vi "Find optimal frequency.vi"(6 "Bottom end of range (GHz) (140.0)":dbl=140.0, 7 "Top end of range (GHz) (141.0)":dbl=141.0, 8 "Find optimal for negative polarization?":bool, 9 "C":dbl, 10 "Fit parameters":T2={"A"=0.572086, "S"=0.0835606, "M1"=140.286, "M2"=140.486}, 11 "Physical constants":T1={"T1e (s)"=0.03, "T1n (s)"=1500.0}) -> (2 "Steady state at optimal frequency":dbl, 3 "Optimal frequency (GHz)":dbl)   [LabVIEW 2018]
uses:
  Fit Parameters.ctl
  Physical Constants.ctl
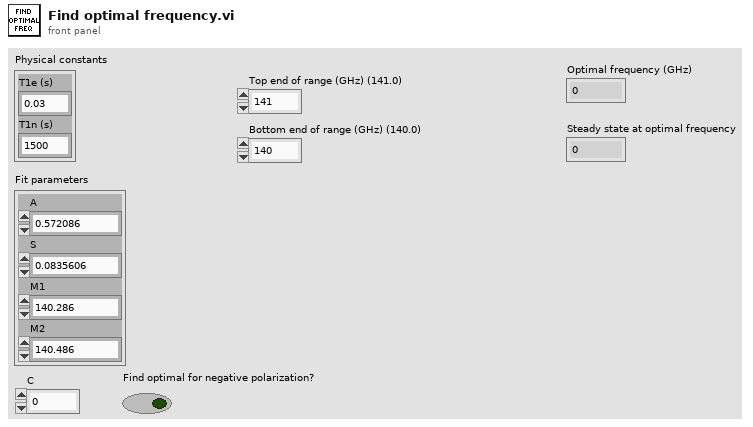
[diagram p1: front panel]
types:
  T1 = typedef "Physical Constants.ctl" = cluster{"T1e (s)":dbl, "T1n (s)":dbl}
  T2 = typedef "Fit Parameters.ctl" = cluster{"A":dbl, "S":dbl, "M1":dbl, "M2":dbl}
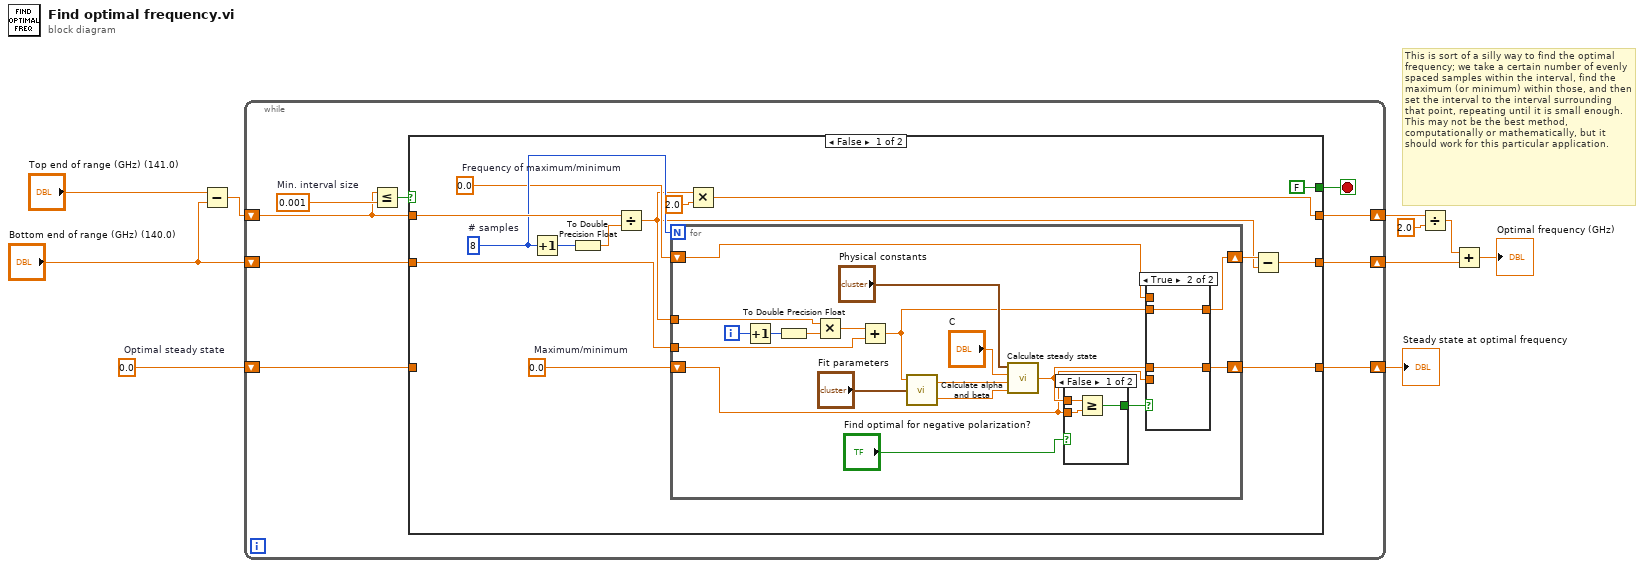
[diagram p0: block diagram]
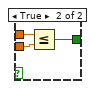
[diagram p3: hidden frame]
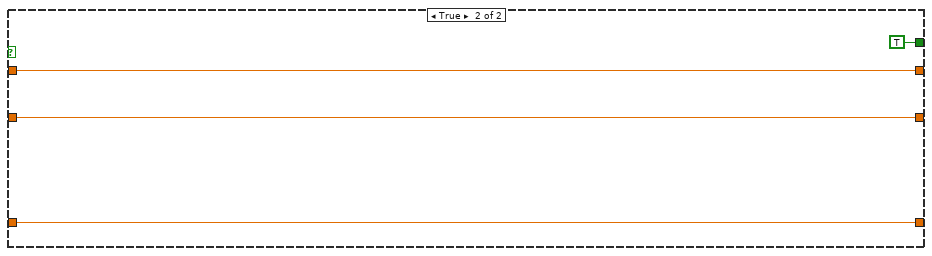
[diagram p4: hidden frame]
diagram:
  w2 = 0.0  # Optimal steady state
  # "This is sort of a silly way to find the optimal frequency; we take a certain number of evenly spaced samples within the interval, find the maximum (or minimum) within those, and then set the interval to the interval surrounding that point, repeating until it is small enough.  This may not be the best method, computationally or mathematically, but it should work for this particular application."
  n1 = Subtract(x="Top end of range (GHz) (141.0)", y="Bottom end of range (GHz) (140.0)") -> (x-y=w8:dbl)
  n2 = while {
    shift-right: [w15] -> w7
    shift-left: w8 -> [w16]
    shift-right: [w13] -> w4
    shift-left: "Bottom end of range (GHz) (140.0)" -> [w14]
    shift-right: [w12] -> w1
    shift-left: w2 -> [w11]
    stop <- w17 stop-if-true
    w19 = 0.001  # Min. interval size
    n3 = Less Or Equal?(x=w16, y=w19) -> (x <= y?=w18:bool)
    n4 = case shown="False" w18 {
      tunnel: [FALSE TRUE] -> w17
      tunnel: w16 -> [w32 w64]
      tunnel: [w27 w64] -> w15
      tunnel: w14 -> [w24 w65]
      tunnel: [w21 w65] -> w13
      tunnel: [w20 w63] -> w12
      tunnel: w11 -> [_ w63]
      frame False {
        w25 = 0.0  # Maximum/minimum
        w26 = 0.0  # Frequency of maximum/minimum
        w29 = 8  # # samples
        n5 = Increment(x=w29) -> (x+1=w30:i32)
        n6 = To Double Precision Float(number=w30) -> (double precision float=w31:dbl)
        n7 = Divide(x=w32, y=w31) -> (x/y=w22:dbl)
        n8 = for {
          N: w29 -> [_]
          tunnel: w22 -> [w51]
          shift-right: [w37] -> w23
          shift-left: w26 -> [w35]
          shift-right: [w36] -> w20
          shift-left: w25 -> [w34]
          tunnel: w24 -> [w39]
          i -> [w49]
          n9 = Increment(x=w49) -> (x+1=w50:i32)
          n10 = To Double Precision Float(number=w50) -> (double precision float=w52:dbl)
          n11 = Multiply(x=w51, y=w52) -> (x*y=w40:dbl)
          n12 = Add(x=w40, y=w39) -> (x+y=w38:dbl)
          n13 = call "Calculate alpha and beta.vi"("Fit parameters"="Fit parameters", "Frequency (GHz)"=w38) -> ("Beta"=w45:dbl, "Alpha"=w46:dbl)  [unwired: 1 in]
          n14 = call "Calculate steady state.vi"("Beta"=w45, "Alpha"=w46, "C"="C", "Physical constants"="Physical constants") -> ("Steady state"=w41:dbl)
          n15 = case shown="False" "Find optimal for negative polarization?" {
            tunnel: w41 -> [w59 w62]
            tunnel: w34 -> [w58 w61]
            tunnel: [w57 w60] -> w42
            frame False {
              n16 = Greater Or Equal?(x=w59, y=w58) -> (x >= y?=w57:bool)
            }
            frame True {
              n17 = Less Or Equal?(x=w62, y=w61) -> (x <= y?=w60:bool)
            }
          }
          n18 = case shown="True" w42 {
            tunnel: w41 -> [_ w55]
            tunnel: w38 -> [_ w56]
            tunnel: [w54 w56] -> w37
            tunnel: [w53 w55] -> w36
            tunnel: w35 -> [w54 _]
            tunnel: w34 -> [w53 _]
            frame False {
            }
            frame True {
            }
          }
        }
        n19 = Multiply(x=w22, y=2.0) -> (x*y=w27:dbl)
        n20 = Subtract(x=w23, y=w22) -> (x-y=w21:dbl)
      }
      frame True {
      }
    }
  }
  "Steady state at optimal frequency" <- w1
  n21 = Divide(x=w7, y=2.0) -> (x/y=w5:dbl)
  n22 = Add(x=w5, y=w4) -> (x+y=→"Optimal frequency (GHz)":dbl)
